vi "filtroColores.vi"(3 "V":dbl, 4 "S":dbl) -> (0 "0, 1":u32, 1 "Color":u32(colorbox))   [LabVIEW 2021]
panel:
  in  "H":dbl
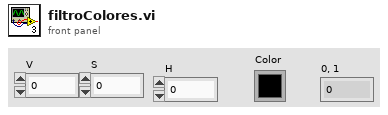
[diagram p1: front panel]
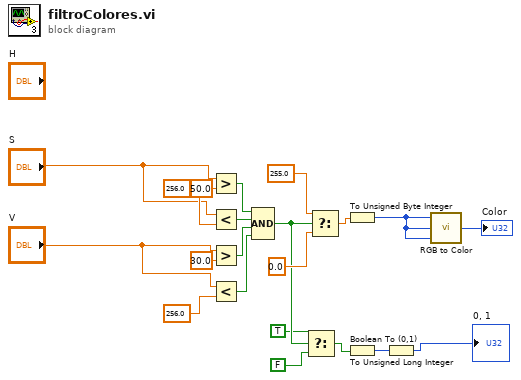
[diagram p0: block diagram]
diagram:
  n1 = Greater?(x="S", y=50.0 ("Smin")) -> (0:w21:bool)
  n2 = Less?(x="S", y=256.0 ("Smax")) -> (x < y?=w20:bool)
  n3 = Greater?(x="V", y=30.0 ("Vmin")) -> (0:w19:bool)
  n4 = Less?(x="V", y=256.0 ("Vmax")) -> (x < y?=w18:bool)
  n5 = Compound Arithmetic op=AND(w21, w20, w19, w18) -> (w6:bool)
  n6 = Select(t=TRUE, s=w6, f=FALSE) -> (s? t:f=w3:bool)
  n7 = Select(t=255.0, s=w6, f=0.0) -> (s? t:f=w10:dbl)
  n8 = To Unsigned Byte Integer(number=w10) -> (unsigned 8bit integer=w9:u8)
  n9 = Boolean To (0,1)(Boolean=w3) -> (0, 1=w2:i16)
  n10 = To Unsigned Long Integer(number=w2) -> (unsigned 32bit integer=→"0, 1":u32)
  n11 = call <vilib>:"RGB to Color.vi"("B"=w9, "G"=w9, "R"=w9) -> ("Color"=→"Color":u32)
